vi "Test Launch Error.vi"(8 "error in":errorcluster, 11 "Test Case In":refnum<class "PreLaunch Error.lvclass">) -> (0 "error out":errorcluster, 3 "Test Case Out":refnum<class "PreLaunch Error.lvclass">)   [LabVIEW 2020, in "PreLaunch Error.lvlib" / "PreLaunch Error.lvclass"]
uses:
  PreLaunch Error.lvclass
  C:/Program Files/National Instruments/LabVIEW 2024/vi.lib/Astemes/LUnit/Test Case.lvclass
  Launch/Launch.lvclass
  C:/Users/J63553/Projects/_LabVIEW Community/actor-framework/Core/ActorFramework/Actor/Actor.lvclass
  Core/ActorFramework/Message Queue/Message Queue.lvclass/Message Queue.ctl
  <vilib>/Astemes/LUnit/Test Case.lvclass/Test Case.ctl
  788af886-0fbf-44a6-b03f-842c545bbad4.vi
  <vilib>/Astemes/LUnit/Append Pass Result.vi
  <vilib>/Astemes/LUnit/Append Fail Result.vi
  788af886-0fbf-44a6-b03f-842c545bbad4.vi/9c5d11cd-9439-4240-a1ee-d9baace9c924.vi
  <vilib>/Astemes/LUnit/Run In UI.vi
  <vilib>/Utility/error.llb/Clear Errors.vi
  Core/ActorFramework/Actor/Actor.lvclass
  Core/ActorFramework/Message Queue/Message Queue.lvclass
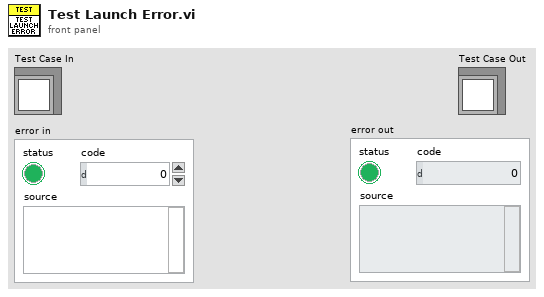
[diagram p1: front panel]
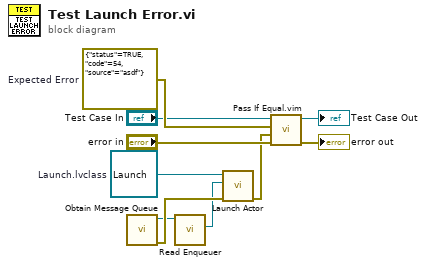
[diagram p0: block diagram]
diagram:
  w7 = errorcluster {"status"=TRUE, "code"=54, "source"="asdf"}  # Expected Error
  w5 = refnum<class "Launch.lvclass"> refnum  # Launch.lvclass
  n1 = call "Obtain Message Queue.vi"() -> ("error out"=w10:errorcluster, "Message Queue"=w4:refnum<class "Message Queue.lvclass">)  [unwired: 10 in]
  n2 = call "Read Enqueuer.vi"("Message Queue"=w4) -> ("Message Enqueuer"=w3:refnum<class "Message Enqueuer.lvclass">)  [unwired: 10 in]
  n3 = call "Launch Actor.vi"("error in (no error)"=w10, "Actor-to-Caller Enqueuer"=w3, "Actor"=w5) -> ("error out"=w6:errorcluster)  [unwired: 7 in, 1 out]
  n4 = call "Pass If Equal.vim"("error in (no error)"="error in", "Actual"=w6, "Expected"=w7, "LUnit Test Case In"="Test Case In") -> ("error out"=→"error out":errorcluster, "LUnit Test Case Out"=→"Test Case Out":refnum<class "PreLaunch Error.lvclass">)  [unwired: 6 in]
